vi "Show In Subpanel.vi"(8 "error in (no error)":errorcluster, 10 "Sub Panel":refnum<vi>, 11 "JQMHCore in":refnum<class "Module.lvclass">) -> (0 "error out":errorcluster, 3 "JQMHCore out":refnum<class "Module.lvclass">)   [LabVIEW 2024, in "Module.lvclass"]
uses:
  Module.lvclass
  Module.lvclass/Module.ctl
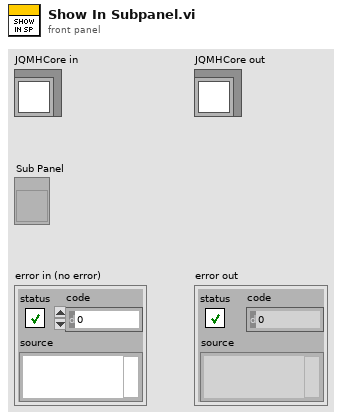
[diagram p1: front panel]
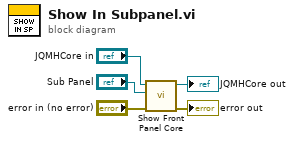
[diagram p0: block diagram]
diagram:
  n1 = call "Show Front Panel Core.vi"("error in (no error)"="error in (no error)", "Data"="Sub Panel", "JQMHCore in"="JQMHCore in") -> ("error out"=→"error out":errorcluster, "JQMHCore out"=→"JQMHCore out":refnum<class "Module.lvclass">)  [unwired: 7 in]
